vi "Configure Voltage.vi"(8 "error in (no error)":errorcluster, 9 "Voltage Level (0.0 V)":dbl format="%.2g", 10 "Preset":i32(ring) items=["Preset1", "Preset2", "Preset3", "Normal Mode"], 11 "VISA resource name":refnum<visa-resource-name>) -> (0 "error out":errorcluster, 3 "VISA resource name out":refnum<visa-resource-name>)   [LabVIEW 2022 SP3, in "BK Precision 9103.lvlib"]
doc: "Configures output voltage level of the power supply."
uses:
  <instrlib>/BK Precision 9103/BK Precision 9103.lvlib
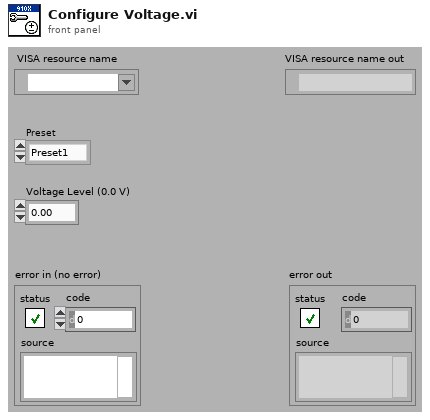
[diagram p1: front panel]
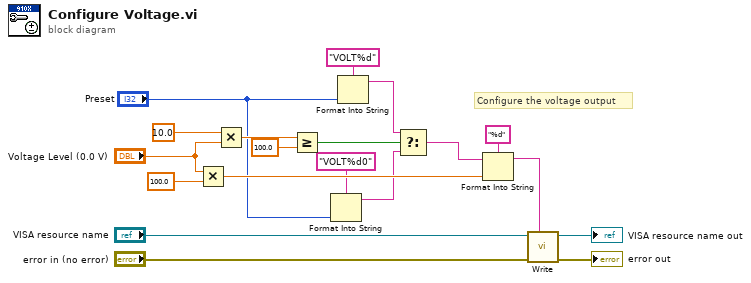
[diagram p0: block diagram]
diagram:
  # "Configure the voltage output"
  n1 = Multiply(x="Voltage Level (0.0 V)", y=100.0) -> (x*y=w12:dbl)
  n2 = Multiply(x=10.0 ("y"), y="Voltage Level (0.0 V)") -> (x*y=w6:dbl)
  n3 = Greater Or Equal?(x=w6, y=100.0) -> (x >= y?=w17:bool)
  n4 = Format Into String(format string="VOLT%d0", "Preset") -> (resulting string=w4:string)  [unwired: 2 in, 1 out]
  n5 = Format Into String(format string="VOLT%d", "Preset") -> (resulting string=w7:string)  [unwired: 2 in, 1 out]
  n6 = Select(t=w7, s=w17, f=w4) -> (s? t:f=w2:string)
  n7 = Format Into String(format string="%d", initial string=w2, w12) -> (resulting string=w11:string)  [unwired: 1 in, 1 out]
  n8 = call <instrlib>:"Write.vi"("Input String"=w11, "error in (no error)"="error in (no error)", "VISA resource name"="VISA resource name") -> ("error out"=→"error out":errorcluster, "VISA resource name out"=→"VISA resource name out":refnum<visa-resource-name>)  [unwired: 6 in, 1 out]
